vi "TW Post-Project-Copying Process - Stage 2.vi"(8 "error in":errorcluster) -> (0 "error out":errorcluster)   [LabVIEW 2021, in "Plugin Generator.lvlib"]
uses:
  Plugin Generator.lvlib
panel:
  in  "Project Name":string
  in  "Project Path":path
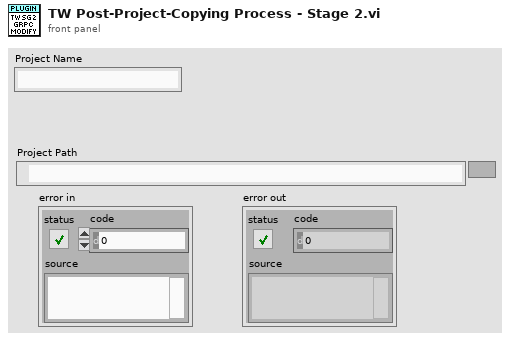
[diagram p1: front panel]
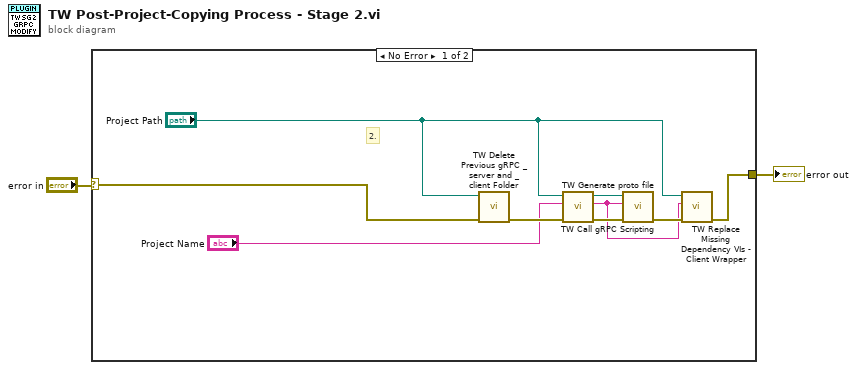
[diagram p0: block diagram]
diagram:
  n1 = case shown="No Error" "error in" {
    selector: "error in" -> [w4 w12]
    tunnel: [w10 w12] -> w2
    frame No Error {
      # "2."
      n2 = call "TW Delete Previous gRPC _server and _client Folder.vi"("error in"=w4, "Project Path"="Project Path") -> ("error out"=w5:errorcluster)  [unwired: 9 in]
      n3 = call "TW Generate proto file.vi"("error in"=w5, "Project Name"="Project Name", "Project Path"="Project Path") -> ("error out"=w9:errorcluster, "gRPC Service Name"=w7:string, "proto File Path"=w8:path)  [unwired: 6 in]
      n4 = call "TW Call gRPC Scripting.vi"("error in"=w9, "gRPC Service Name"=w7, "proto File Path"=w8) -> ("error out"=w11:errorcluster)  [unwired: 8 in]
      n5 = call "TW Replace Missing Dependency VIs - Client Wrapper.vi"("error in"=w11, "gRPC Service Name"=w7, "Project Path"="Project Path") -> ("error out"=w10:errorcluster)  [unwired: 8 in]
    }
    frame Error {
    }
  }
  "error out" <- w2
